vi "PSD calculation and fitting.vi"() -> ()   [LabVIEW 2014]
uses:
  <vilib>/Analysis/2dsp.llb/1D Auto Correlation (DBL).vi
  <vilib>/Analysis/2dsp.llb/Real FFT.vi
  <vilib>/Utility/file.llb/Read From Spreadsheet File (DBL).vi
  <vilib>/gmath/NumericalOptimization/Nonlinear Curve Fit LM formula string.vi
  <vilib>/Analysis/NI_AALPro.lvlib
  <vilib>/gmath/NI_Gmath.lvlib
panel:
  in  "termination":cluster{"max iteration":i32, "tolerance":dbl}={"max iteration"=200, "tolerance"=1e-08}
  out "best fit parameters":dbl[](array[numeric])
  in  "initial parameters":dbl[](array[numeric])
  out "FFT method Graph 2":cluster{dbl[], dbl[]}(graph)
  out "Waveform Graph 2":dbl[](graph)
  out "size(s) 2":i32
  out "Auto PSD fit":dbl[](array[numeric]) format="%.4f"
  out "subarray":dbl[](array[numeric])
  out "AutoCorr":dbl[](array[numeric])
  out "Waveform Graph":dbl[](graph)
  out "ac 2":i32
  out "ac":i32
  out "avg. #":dbl
  in  "sampling frequency (Hz)":i32
  out "size(s)":i32
  out "FT method":dbl[](array[numeric]) format="%#_6f"
  in  "Tab Control":T1(tab)
  out "(no avg)FFT method Graph":cluster{dbl[], dbl[]}(graph)
  out "FFT method Graph":cluster{dbl[], dbl[]}(graph)
  out "XY Graph 3":cluster{dbl[], "Array":dbl[]}[](graph)
  out "AutoCorrelation method":cluster{dbl[], "Array":dbl[]}[](graph)
  out "AutoPSD":cluster{dbl[], "Array":dbl[]}[](graph)
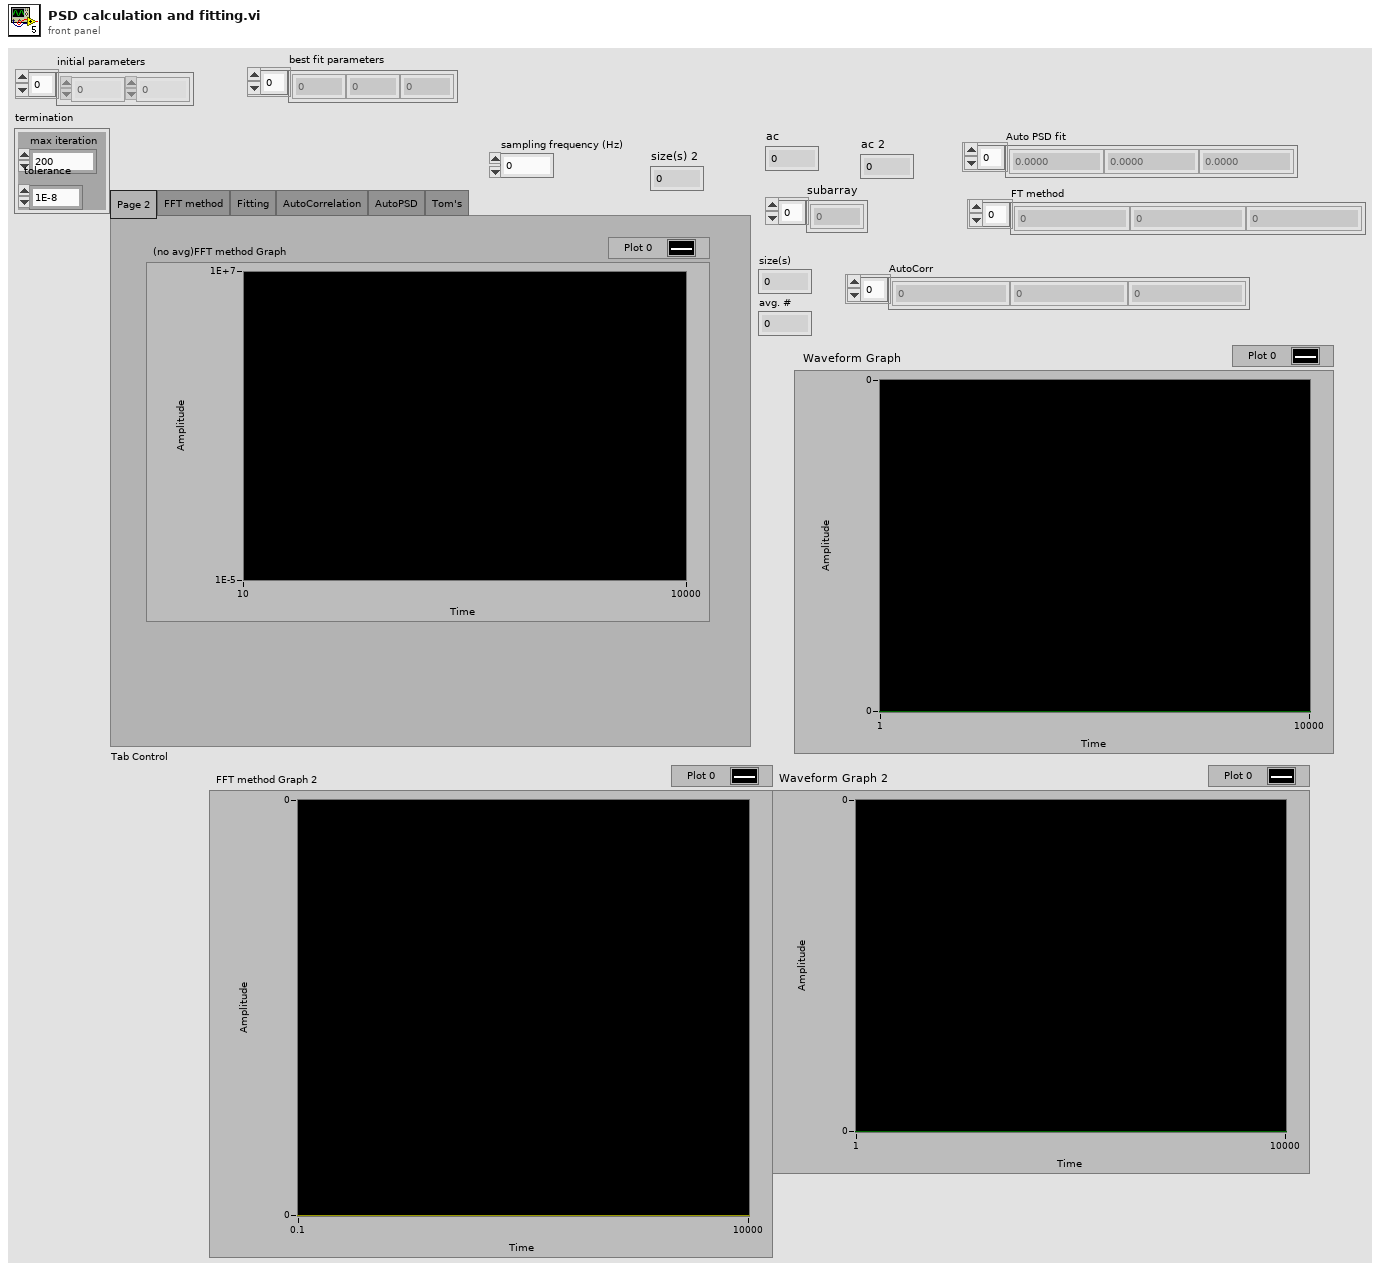
[diagram p1: front panel]
types:
  T1 = enum32{"Page 2", "FFT method", "Fitting", "AutoCorrelation", "AutoPSD", "Tom's"}
  T2 = cluster{"model":string, "Parameters":string[], "x":string}
  T3 = enum32{"Vrms", "Vpk", "Vrms^2", "Vpk^2", "Vrms/rtHz", "Vpk/rtHz", "Vrms^2/Hz", "Vpk^2/Hz"}
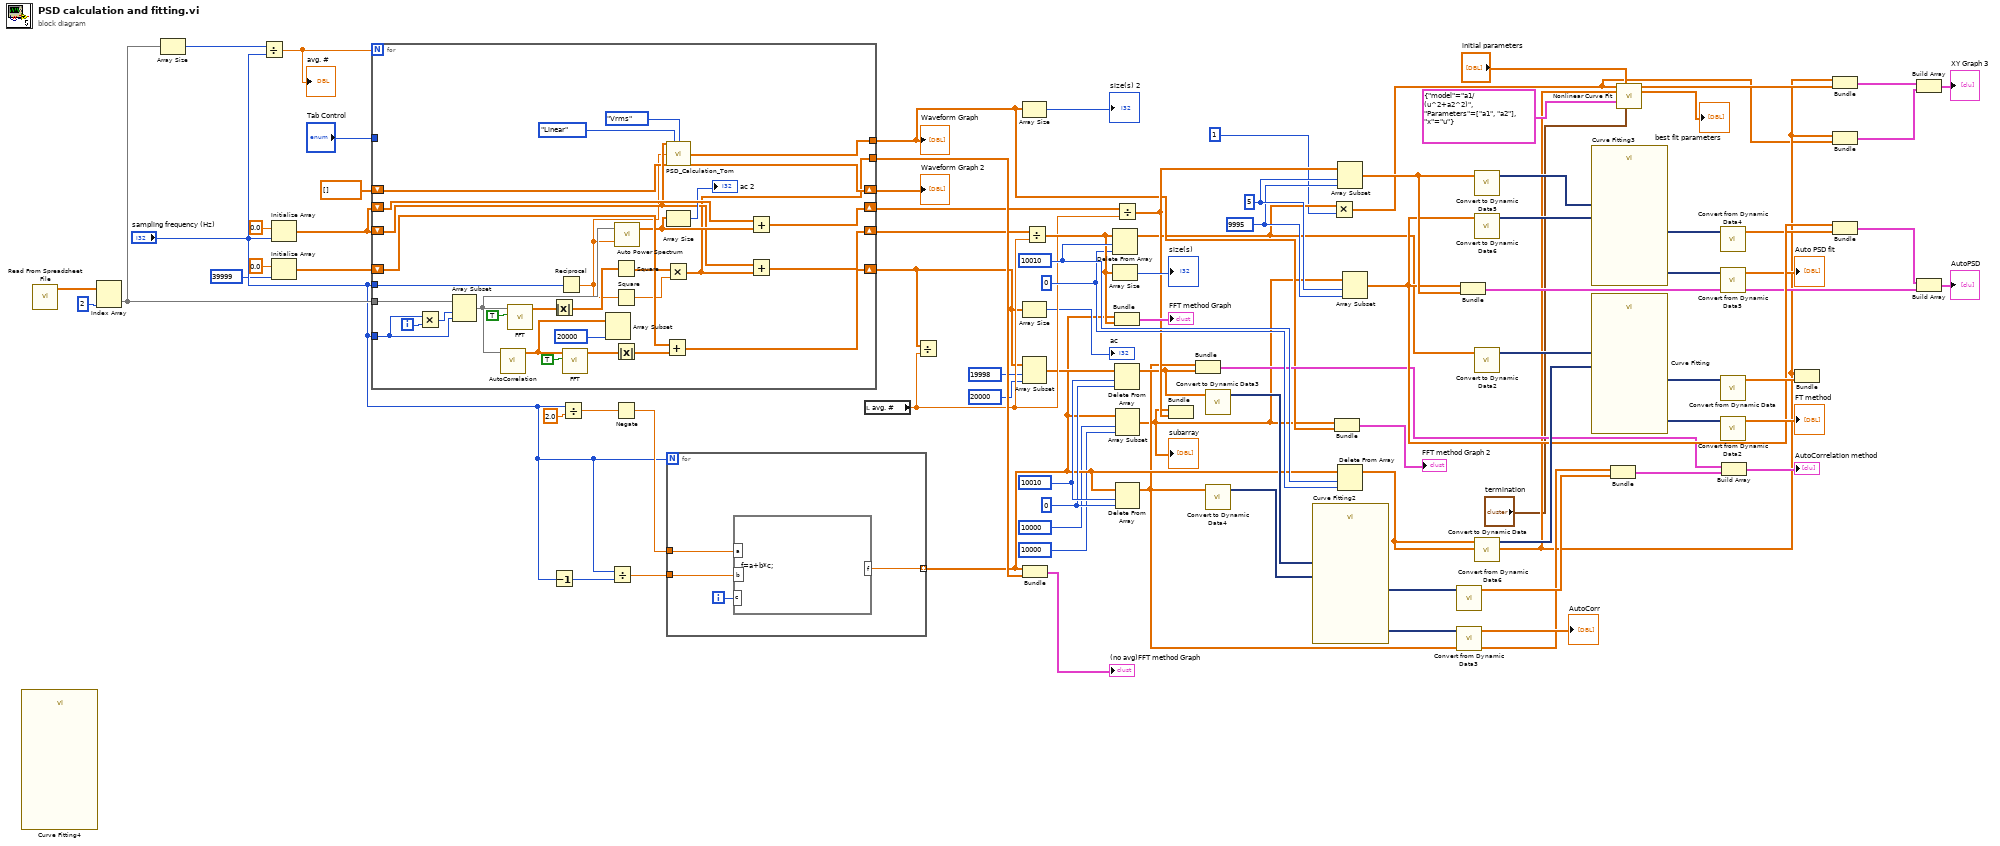
[diagram p0: block diagram]
diagram:
  w37 = 5 ("index")
  w36 = 9995 ("length")
  w47 = 10010 ("length")
  w46 = 0 ("index")
  w63 = 10010 ("length")
  w59 = 0 ("index")
  n1 = call "Curve Fitting4"() -> ()  [unwired: 7 in, 5 out]
  n2 = call-poly <vilib>:"Read From Spreadsheet File.vi"() -> ("all rows"=w86:dbl[][])  [unwired: 7 in, 4 out]
  n3 = Index Array(array=w86, index (col)=2 ("disabled index (col)")) -> (element=w72:dbl[])  [unwired: 1 in]
  n4 = Array Size(array=w72) -> (size(s)=w80:i32)
  n5 = Divide(x=w80, y="sampling frequency (Hz)") -> (x/y=w79:dbl)
  "avg. #" <- w79
  n6 = Initialize Array(0.0 ("element"), "sampling frequency (Hz)") -> (w52:dbl[])
  n7 = Initialize Array(0.0 ("element"), 39999 ("dimension size")) -> (w51:dbl[])
  n8 = for {
    N: w79 -> [_]
    tunnel: w72 -> [w117]
    tunnel: "sampling frequency (Hz)" -> [w113]
    tunnel: [w87] -> w81
    shift-right: [w110] -> w75
    shift-left: w52 -> [w96]
    tunnel: "Tab Control" -> [_]
    shift-right: [w106] -> w49
    shift-left: w51 -> [w108]
    tunnel: "sampling frequency (Hz)" -> [w104]
    shift-right: [w102] -> w71
    shift-left: w52 -> [w103]
    shift-right: [w95] -> w14
    shift-left: dbl[] [] ("Power Spectrum (V^2 rms) Out") -> [w94]
    tunnel: [w93] -> w13
    i -> [w114]
    n9 = Multiply(x=w113, y=w114) -> (x*y=w116:i32)
    n10 = Array Subset(array=w117, index=w116, length=w113) -> (w105:dbl[])
    n11 = call-poly <vilib>:"AutoCorrelation.vi"("X"=w105) -> ("Rxx"=w98:dbl[])  [unwired: 9 in, 1 out]
    n12 = call-poly <vilib>:"FFT.vi"("shift?"=TRUE, "X"=w105) -> ("FFT {X}"=w112:cdb[])  [unwired: 8 in, 1 out]
    n13 = Absolute Value(x=w112) -> (abs(x)=w111:dbl[])
    n14 = Reciprocal(x=w104) -> (1/x=w89:dbl)
    n15 = call-poly <vilib>:"FFT.vi"("shift?"=TRUE, "X"=w98) -> ("FFT {X}"=w99:cdb[])  [unwired: 8 in, 1 out]
    n16 = Array Subset(array=w98, length=20000) -> ()  [unwired: 1 in, 1 out]
    n17 = Square(x=w111) -> (x^2=w90:dbl[])
    n18 = Square(x=w89) -> (x^2=w88:dbl)
    n19 = Absolute Value(x=w99) -> (abs(x)=w107:dbl[])
    n20 = call <vilib>:"Auto Power Spectrum.vi"("dt"=w89, "Signal (V)"=w105) -> ("Power Spectrum (V^2 rms)"=w97:dbl[])  [unwired: 1 out]
    n21 = Add(x=w108, y=w107) -> (x+y=w106:dbl[])
    n22 = Multiply(x=w90, y=w88) -> (x*y=w87:dbl[])
    n23 = call "PSD_Calculation_Tom.vi"("Scaled Data 1D"=w96, "log/linear"=enum16{"Linear", "dB", "dBm"}."Linear", "display unit"=T3."Vrms", "dt"=w89, "Power Spectrum (V^2 rms)"=w94) -> ("Avg PSD"=w93:dbl[], "Power Spectrum (V^2 rms) Out"=w95:dbl[])  [unwired: 5 in, 4 out]
    n24 = Array Size(array=w97) -> (size(s)=→"ac 2":i32)
    n25 = Add(x=w103, y=w97) -> (x+y=w102:dbl[])
    n26 = Add(x=w96, y=w87) -> (x+y=w110:dbl[])
  }
  "Waveform Graph" <- w13
  "Waveform Graph 2" <- w14
  n27 = Decrement(x="sampling frequency (Hz)") -> (x-1=w82:i32)
  n28 = Divide(x="sampling frequency (Hz)", y=2.0) -> (x/y=w83:dbl)
  n29 = Divide(x="sampling frequency (Hz)", y=w82) -> (x/y=w77:dbl)
  n30 = Negate(x=w83) -> (-x=w78:dbl)
  n31 = for {
    N: "sampling frequency (Hz)" -> [_]
    tunnel: w78 -> [w121]
    tunnel: w77 -> [w120]
    tunnel: [w118] -> w40 mode=indexing
    i -> [w119]
    n32 = formula code="f=a+b*c;"("a"=w121, "b"=w120, "c"=w119) -> ("f"=w118:dbl)
  }
  n33 = local read "avg. #"() -> (w56:dbl)
  n34 = Divide(x=w49, y=w56) -> ()  [unwired: 1 out]
  n35 = Array Size(array=w13) -> (size(s)=→"size(s) 2":i32)
  n36 = Array Size(array=w49) -> (size(s)=→"ac":i32)
  n37 = Array Subset(array=w49, index=19998, length=20000) -> (w45:dbl[])
  n38 = Bundle(w40, w81) -> (→"(no avg)FFT method Graph":cluster{dbl[], dbl[]})  [unwired: 1 in]
  n39 = Divide(x=w75, y=w56) -> (x/y=w62:dbl[])
  n40 = Delete From Array(array=w62, length=w63, index=w59) -> (array with subset deleted=w4:dbl[])  [unwired: 1 out]
  n41 = Array Size(array=w62) -> (size(s)=→"size(s)":i32)
  n42 = Bundle(w40, w62) -> (→"FFT method Graph":cluster{dbl[], dbl[]})  [unwired: 1 in]
  n43 = Delete From Array(array=w45, length=w47, index=w46) -> (array with subset deleted=w22:dbl[])  [unwired: 1 out]
  n44 = Divide(x=w71, y=w56) -> (x/y=w35:dbl[])
  n45 = Array Subset(array=w40, index=10000, length=10000) -> (w12:dbl[])
  "subarray" <- w12
  n46 = Delete From Array(array=w40, length=w47, index=w46) -> (array with subset deleted=w21:dbl[])  [unwired: 1 out]
  n47 = Bundle(w12, w35) -> ()  [unwired: 1 in, 1 out]
  n48 = Bundle(w21, w22) -> (w20:cluster{dbl[], dbl[]})  [unwired: 1 in]
  n49 = call "Convert to Dynamic Data3"("Array"=w22) -> ("Dynamic Data Type"=w44:dynamicdata)  [unwired: 3 in]
  n50 = call "Convert to Dynamic Data4"("Array"=w21) -> ("Dynamic Data Type"=w43:dynamicdata)  [unwired: 3 in]
  n51 = call "Curve Fitting2"("Locations"=w43, "Signals"=w44) -> ("best fit"=w25:dynamicdata, "non-linear coefficients"=w42:dynamicdata)  [unwired: 5 in, 3 out]
  n52 = Multiply(x=w4, y=1) -> (x*y=w1:dbl[])
  n53 = Bundle(w12, "Avg PSD"=w13) -> (→"FFT method Graph 2":cluster{dbl[], "Avg PSD":dbl[]})  [unwired: 1 in]
  n54 = Array Subset(array=w35, index=w37, length=w36) -> (w32:dbl[])
  n55 = Delete From Array(array=w40, length=w63, index=w59) -> (array with subset deleted=w6:dbl[])  [unwired: 1 out]
  n56 = Array Subset(array=w12, index=w37, length=w36) -> (w31:dbl[])
  n57 = call "Convert from Dynamic Data6"("Dynamic Data Type"=w25) -> ("Array"=w24:dbl[])  [unwired: 3 in]
  n58 = call "Convert from Dynamic Data3"("Dynamic Data Type"=w42) -> ("Array"=→"AutoCorr":dbl[])  [unwired: 3 in]
  n59 = Bundle(w31, w32) -> (w17:cluster{dbl[], dbl[]})  [unwired: 1 in]
  n60 = call "Convert to Dynamic Data5"("Array"=w32) -> ("Dynamic Data Type"=w34:dynamicdata)  [unwired: 3 in]
  n61 = call "Convert to Dynamic Data6"("Array"=w31) -> ("Dynamic Data Type"=w33:dynamicdata)  [unwired: 3 in]
  n62 = call "Convert to Dynamic Data2"("Array"=w4) -> ("Dynamic Data Type"=w69:dynamicdata)  [unwired: 3 in]
  n63 = call "Convert to Dynamic Data"("Array"=w6) -> ("Dynamic Data Type"=w70:dynamicdata)  [unwired: 3 in]
  n64 = call "Curve Fitting3"("Locations"=w33, "Signals"=w34) -> ("best fit"=w30:dynamicdata, "non-linear coefficients"=w27:dynamicdata)  [unwired: 5 in, 3 out]
  n65 = call "Curve Fitting"("Locations"=w70, "Signals"=w69) -> ("best fit"=w58:dynamicdata, "non-linear coefficients"=w65:dynamicdata)  [unwired: 5 in, 3 out]
  n66 = Bundle(w21, "Array"=w24) -> (w23:cluster{dbl[], "Array":dbl[]})  [unwired: 1 in]
  n67 = call-poly <vilib>:"Nonlinear Curve Fit.vi"("Y"=w1, "initial parameters"="initial parameters", "X"=w6, "model description"=T2 {"model"="a1/(u^2+a2^2)", "Parameters"=["a1", "a2"], "x"="u"}, "termination"="termination") -> ("best nonlinear fit"=w7:dbl[], "best fit parameters"=→"best fit parameters":dbl[])  [unwired: 6 in, 3 out]
  n68 = call "Convert from Dynamic Data4"("Dynamic Data Type"=w30) -> ("Array"=w29:dbl[])  [unwired: 3 in]
  n69 = call "Convert from Dynamic Data5"("Dynamic Data Type"=w27) -> ("Array"=→"Auto PSD fit":dbl[])  [unwired: 3 in]
  n70 = call "Convert from Dynamic Data"("Dynamic Data Type"=w58) -> ("Array"=w68:dbl[])  [unwired: 3 in]
  n71 = call "Convert from Dynamic Data2"("Dynamic Data Type"=w65) -> ("Array"=→"FT method":dbl[])  [unwired: 3 in]
  n72 = Build Array(w20, w23) -> (→"AutoCorrelation method":cluster{dbl[], "Array":dbl[]}[])
  n73 = Bundle(w6, "Array"=w68) -> ()  [unwired: 1 in, 1 out]
  n74 = Bundle(w6, "best nonlinear fit"=w7) -> (w5:cluster{dbl[], "best nonlinear fit":dbl[]})  [unwired: 1 in]
  n75 = Bundle(w6, w1) -> (w60:cluster{dbl[], dbl[]})  [unwired: 1 in]
  n76 = Bundle(w31, "Array"=w29) -> (w18:cluster{dbl[], "Array":dbl[]})  [unwired: 1 in]
  n77 = Build Array(w5, w60) -> (→"XY Graph 3":cluster{dbl[], "best nonlinear fit":dbl[]}[])
  n78 = Build Array(w18, w17) -> (→"AutoPSD":cluster{dbl[], "Array":dbl[]}[])
